vi "GetBlockSettingsFile.vi"(5 "# Cycles":i16=20, 6 "target set #":i16, 7 "Block":T1(array[cluster])) -> (0 "Completed list?":bool, 2 "# target sets":i16, 3 "Settings file":path)   [LabVIEW 2010]
doc: "The purpose of this vi is to determine, based on the number of completed target sets, where in the block list we currently are, and whether we need to instantiate new settings (i.e., because we have crossed from one block to another)."
panel:
  out "total sets":u16
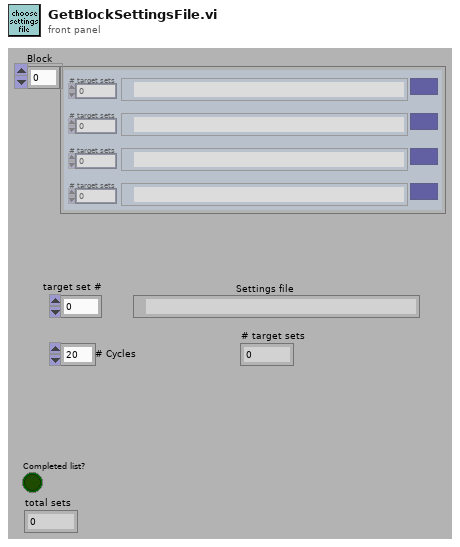
[diagram p1: front panel]
types:
  T1 = cluster{"Settings file":path, "# target sets":u16}[]
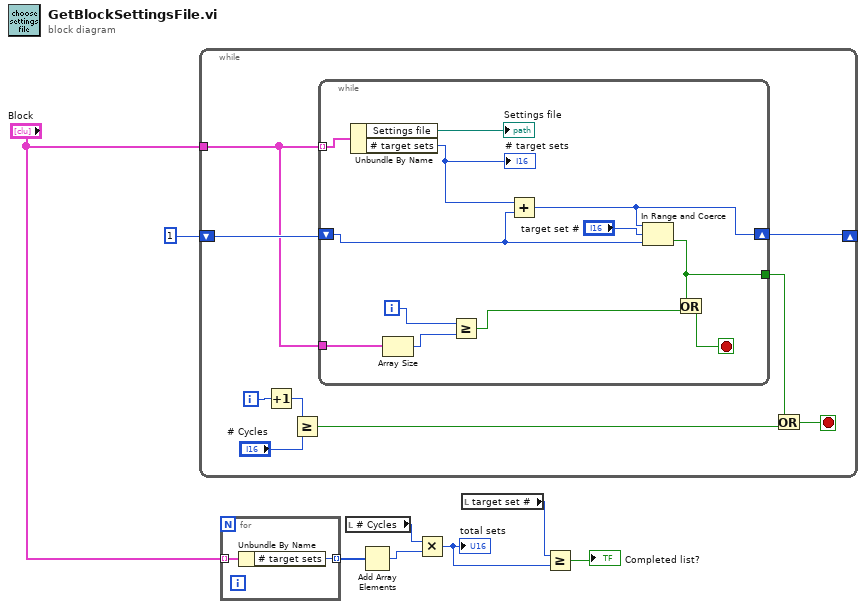
[diagram p0: block diagram]
diagram:
  n1 = while {
    shift-right: [w16] -> _
    shift-left: i16 1 ("# target sets") -> [w17]
    tunnel: "Block" -> [w9]
    i -> [w13]
    stop <- w14 stop-if-true
    n2 = Increment(x=w13) -> (x+1=w11:i32)
    n3 = Greater Or Equal?(x=w11, y="# Cycles") -> (x >= y?=w10:bool)
    n4 = while {
      tunnel: w9 -> [w21] mode=indexing
      shift-right: [w22] -> w16
      shift-left: w17 -> [w25]
      tunnel: [w26] -> w15
      tunnel: w9 -> [w20]
      i -> [w18]
      stop <- w27 stop-if-true
      n5 = Unbundle By Name(w21) -> ("Settings file"=→"Settings file":path, "# target sets"=w23:u16)
      "# target sets" <- w23
      n6 = Array Size(array=w20) -> (size(s)=w19:i32)
      n7 = Greater Or Equal?(x=w18, y=w19) -> (x >= y?=w24:bool)
      n8 = Add(x=w23, y=w25) -> (x+y=w22:u16)
      n9 = In Range and Coerce(upper limit=w22, x="target set #", lower limit=w25) -> (In Range?=w26:bool)  [unwired: 1 out]
      n10 = Or(x=w26, y=w24) -> (x .or. y?=w27:bool)
    }
    n11 = Or(x=w15, y=w10) -> (x .or. y?=w14:bool)
  }
  n12 = for {
    tunnel: "Block" -> [w31] mode=indexing
    tunnel: [w30] -> w6 mode=indexing
    n13 = Unbundle By Name(w31) -> ("# target sets"=w30:u16)
  }
  n14 = local read "# Cycles"() -> (w5:i16)
  n15 = Add Array Elements(numeric array=w6) -> (sum=w4:u16)
  n16 = Multiply(x=w5, y=w4) -> (x*y=w1:u16)
  "total sets" <- w1
  n17 = local read "target set #"() -> (w2:i16)
  n18 = Greater Or Equal?(x=w2, y=w1) -> (x >= y?=→"Completed list?":bool)
